vi "udp.ip.reader.ip.vi"() -> ()   [LabVIEW 2020]
uses:
  <instrlib>/_niInstr/Network/Types/v1/IPv4 Address.ctl
  <instrlib>/_niInstr/Network/Types/v1/MAC Address.ctl
  <vilib>/Platform/TimedLoop/XDataNode/timing_clust.ctl
  <vilib>/Platform/TimedLoop/XDataNode/nitl_modes.ctl
  <vilib>/Platform/TimedLoop/XDataNode/wakeup.ctl
  <vilib>/rvi/Emulation/niFpgaSctlEmulationGetInTimedLoop.vi
  <vilib>/rvi/Emulation/niFpgaEmulationReportErrorSimple.vi
  <vilib>/rvi/Emulation/niFpgaGetClockAttributes.vi
  <vilib>/rvi/Emulation/niFpgaCriticalErrorInLSC.vi
  <vilib>/Platform/TimedLoop/XDataNode/XDataNode.xnode
  <vilib>/Platform/TimedLoop/XDataNode/XDNodeRunTimeDep.lvlib
  <instrlib>/_niInstr/Network/Types/v1/niInstr Network Types v1.lvlib
panel:
  out "udp_byte_enable":bool
  out "udp_data valid_out":bool
  out "udp_data_out":u8
  in  "MAC Address":T1=[176, 197, 84, 255, 244, 135] format="%.0x"
  in  "IP Address":T2=[176, 197, 84, 255]
  in  "Dest Port":u16
  in  "end_of_frame":bool
  in  "data_valid":bool
  in  "data":u8
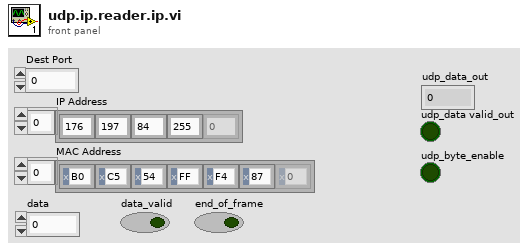
[diagram p1: front panel]
types:
  T1 = typedef "niInstr Network Types v1.lvlib/MAC Address.ctl" = u8[]
  T2 = typedef "niInstr Network Types v1.lvlib/IPv4 Address.ctl" = u8[]
  T3 = typedef "XDNodeRunTimeDep.lvlib/timing_clust.ctl" = cluster{"Expected End [f-1]":u64, "Actual End [f-1]":u64, "Finished Late? [f-1]":bool, "Expected End [i-1]":u64, "Actual End [i-1]":u64, "Finished Late? [i-1]":bool, "Expected Start [i]":u64, "Actual Start [i]":u64, "Expected Start [f]":u64, "Actual Start [f]":u64, "Source Name":string, "Structure Name":string, "Period":i64, "Deadline":i64, "Offset":i64, "Start":i64, "Priority":i32, "Timeout":i32, "Mode":T4, "Wakeup Reason":T5, "Error":errorcluster, "Source Type":string, "Secondary Source Type":string, "Global End Time":u64, "Global Start Time":u64, "Frame Duration":u64, "Iteration Duration":u64, "Assigned CPU":i32, "I/O Scan Engine Mode":u32}
  T4 = typedef "XDNodeRunTimeDep.lvlib/nitl_modes.ctl" = enum32{"No Change", "Process missed periods, maintain original phase", "Discard missed periods, maintain original phase", "Process missed periods, ignore original phase", "Discard missed periods, ignore original phase"}
  T5 = typedef "XDNodeRunTimeDep.lvlib/wakeup.ctl" = enum32{"Normal", "Aborted", "Asynchronous wakeup", "Timing source error", "Timed loop error", "Timeout"}
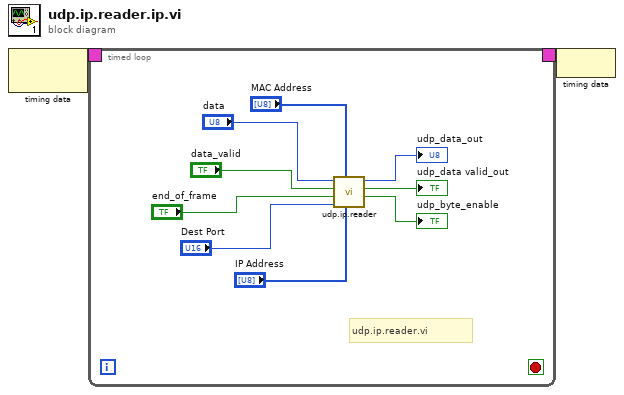
[diagram p0: block diagram]
diagram:
  n1 = node-c288() -> (w2:T3)  [unwired: 1 in]
  n2 = timed-loop {
    timing: w2 -> [_]
    timing-out: [_] -> w1
    stop <- _ stop-if-true
    # "udp.ip.reader.vi"
    n3 = call "udp.ip.reader.vi"("IP Address"="IP Address", "MAC Address"="MAC Address", "Dest Port"="Dest Port", "end_of_frame"="end_of_frame", "data_valid"="data_valid", "data"="data") -> ("udp_byte_enable"=→"udp_byte_enable":bool, "udp_data valid_out"=→"udp_data valid_out":bool, "udp_data_out"=→"udp_data_out":u8)  [unwired: 3 in]
  }
  n4 = node-c288(w1) -> ()
